vi "AH2500.SINGLE.vi"(8 "error in (no error)":errorcluster, 11 "VISA resource name":refnum<visa-resource-name>) -> (0 "error out":errorcluster, 2 "Measurement":T1, 3 "VISA resource name out":refnum<visa-resource-name>)   [LabVIEW 2019, in "Inst.AH2500.lvclass"]
uses:
  Inst.AH2500.lvclass
  Typedefs/Inst.AH2500.getAll--Cluster.ctl
panel:
  out "read buffer":string
  # "Do a single measurement"
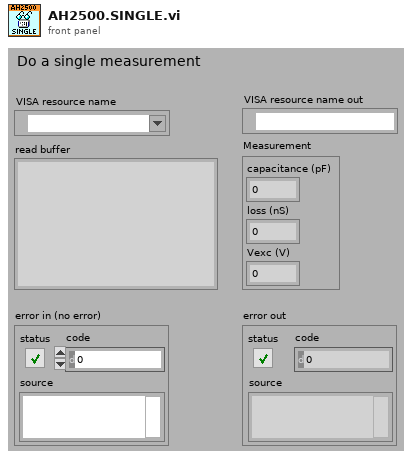
[diagram p1: front panel]
types:
  T1 = typedef "Inst.AH2500.lvclass/Inst.AH2500.getAll--Cluster.ctl" = cluster{"capacitance (pF)":dbl, "loss (nS)":dbl, "Vexc (V)":dbl}
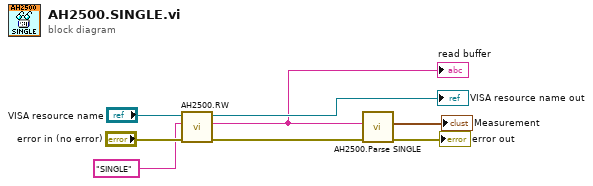
[diagram p0: block diagram]
diagram:
  n1 = call "AH2500.RW.vi"("error in (no error)"="error in (no error)", "write buffer"="SINGLE", "VISA Refnum in"="VISA resource name") -> ("error out"=w3:errorcluster, "read buffer"=w1:string, "VISA Refnum out"=→"VISA resource name out":refnum<visa-resource-name>)  [unwired: 6 in]
  "read buffer" <- w1
  n2 = call "AH2500.Parse SINGLE.vi"("error in"=w3, "read buffer"=w1) -> ("error out"=→"error out":errorcluster, "Measurement"=→"Measurement":T1)  [unwired: 8 in]
